vi "GetElements(Multiple).vi"(7 "Qualified Name":string, 8 "error in (no error)":errorcluster, 10 "keys":string[](array[string]), 11 "ConfigManager.Text in":refnum<class "ConfigManager.Text.lvclass">) -> (0 "error out":errorcluster, 1 "Found":bool[](array[boolean]), 2 "Values":string[](array[string]), 3 "ConfigManager.Text out":refnum<class "ConfigManager.Text.lvclass">)   [LabVIEW 2013, in "CfgManager.Text.lvlib" / "ConfigManager.Text.lvclass"]
uses:
  ConfigManager.Text.lvclass
  ConfigManager.Text.lvclass/ConfigManager.Text.ctl
  Response - cluster.ctl
  Query -- cluster.ctl
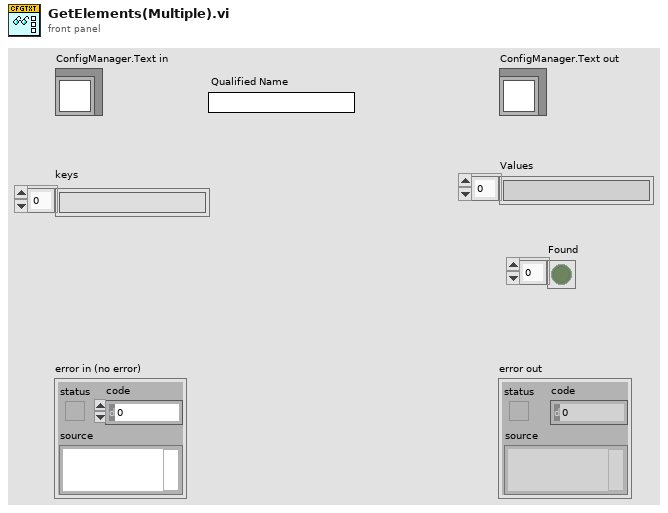
[diagram p1: front panel]
types:
  T1 = typedef "CfgManager.Text.lvlib/ConfigManager.Text.lvclass/Query -- cluster.ctl" = cluster{"Qualified Name":string[], "Keys":string[]}
  T2 = typedef "CfgManager.Text.lvlib/ConfigManager.Text.lvclass/Response - cluster.ctl" = cluster{"Section":string[], "Keys":string[], "Values":string[], "Found":bool[]}
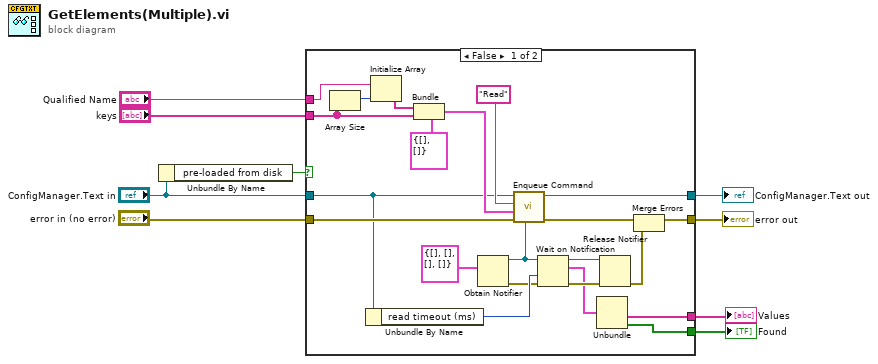
[diagram p0: block diagram]
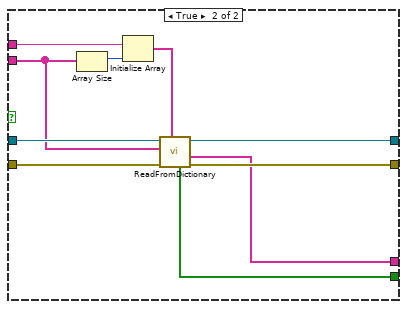
[diagram p2: hidden frame]
diagram:
  n1 = Unbundle By Name("ConfigManager.Text in") -> ("pre-loaded from disk"=w9:bool)
  n2 = case shown="False" w9 {
    tunnel: [w24 w40] -> w3
    tunnel: [w15 w36] -> w1
    tunnel: [w14 w37] -> w2
    tunnel: [w10 w38] -> w7
    tunnel: "Qualified Name" -> [w17 w34]
    tunnel: "error in (no error)" -> [w13 w41]
    tunnel: "keys" -> [w19 w33]
    tunnel: "ConfigManager.Text in" -> [w11 w39]
    frame False {
      n3 = Array Size(array=w19) -> (size(s)=w18:i32)
      n4 = Unbundle By Name(w11) -> ("read timeout (ms)"=w27:i32)
      n5 = Initialize Array(w17, w18) -> (w16:string[])
      n6 = Bundle(cluster=T1 {"Qualified Name"=[], "Keys"=[]} ("Query"), "Qualified Name"=w16, "Keys"=w19) -> (w20:T1)
      n7 = Obtain Notifier(notification data type=T2 {"Section"=[], "Keys"=[], "Values"=[], "Found"=[]} ("response")) -> (notifier out=w22:refnum<notifier>, error out=w26:errorcluster)  [unwired: 3 in, 1 out]
      n8 = call "Enqueue Command.vi"("query notifier"=w22, "error in (no error)"=w13, "args"=w20, "command"="Read", "ConfigManager.Text in"=w11) -> ("error out"=w12:errorcluster, "ConfigManager.Text out"=w10:refnum<class "ConfigManager.Text.lvclass">)  [unwired: 4 in, 1 out]
      n9 = Wait on Notification(notifier=w22, timeout in ms (-1)=w27, error in (no error)=w26) -> (notifier out=w29:refnum<notifier>, notification=w23:T2, error out=w28:errorcluster)  [unwired: 1 in, 1 out]
      n10 = Unbundle(w23) -> ("Values"=w14:string[], "Found"=w15:bool[])  [unwired: 2 out]
      n11 = Release Notifier(notifier=w29, error in (no error)=w28) -> (error out=w25:errorcluster)  [unwired: 1 in, 2 out]
      n12 = Merge Errors(w12, w25) -> (w24:errorcluster)
    }
    frame True {
      n13 = Array Size(array=w33) -> (size(s)=w35:i32)
      n14 = Initialize Array(w34, w35) -> (w32:string[])
      n15 = call "ReadFromDictionary.vi"("Section"=w32, "error in (no error)"=w41, "Keys"=w33, "ConfigManager.Text in"=w39) -> ("error out"=w40:errorcluster, "Values"=w37:string[], "ConfigManager.Text out"=w38:refnum<class "ConfigManager.Text.lvclass">, "Found"=w36:bool[])  [unwired: 2 in, 2 out]
    }
  }
  "error out" <- w3
  "ConfigManager.Text out" <- w7
  "Values" <- w2
  "Found" <- w1
